vi "Teleop.vi"(10 "Match Info":T2={"Autonomous Elapsed Seconds"=0.0, "TeleOp Elapsed Seconds"=0.0, "Disabled Elapsed Seconds"=0.0, "Visited Autonomous"=FALSE, "Visited TeleOp"=FALSE, "Visited Disabled"=FALSE, "Autonomous Settings"={"Autonomous Style"=enum."Independent", "VI Refnum"=refnum}}, 11 "Call Context":T3) -> ()   [LabVIEW 2016]
doc: "This VI is called for each TeleOp packet received from the DS where the robot is not disabled. It is often used to read from the joysticks and update I/O or to update setpoints for timed control loops. It should complete and return within 20 milliseconds or it may miss DS packets."
uses:
  <vilib>/Rock Robotics/WPI/DriverStation/WPI_DriverStationDerivedRobotMode.ctl
  <vilib>/Rock Robotics/WPI/DriverStation/WPI_DriverStationMatch Info.ctl
  <vilib>/Rock Robotics/WPI/ThirdParty/CanMotor/TalonSRX/WPI_CANTalonSRX_GlobalStatus.ctl
  <vilib>/Rock Robotics/WPI/Relay/WPI_RelayValue.ctl
  <vilib>/Rock Robotics/Network Tables/NT Read Number.vi
  <vilib>/Rock Robotics/Network Tables/NT Read Boolean.vi
  <vilib>/Rock Robotics/WPI/Utilities/WPI_GetSetVariantRefNum.vi
  <vilib>/Rock Robotics/Network Tables/NT Write Boolean Array.vi
  <vilib>/Rock Robotics/Network Tables/NT Write Numeric Array.vi
  <vilib>/Rock Robotics/WPI/Ultrasonic/WPI_SonarMB1010DigitalRefNum Registry Get.vi
  <vilib>/Rock Robotics/WPI/Ultrasonic/WPI_SonarMB1010DigitalGetRange.vi
  <vilib>/Rock Robotics/Network Tables/NT Write Number.vi
  <vilib>/gmath/NI_Gmath.lvlib
panel:
  in  "Low Speed Divisor":dbl format="%#_13g"
  out "Encoder Position 2":dbl
  out "Talon SRX Status":T1
  out "Encoder Position":dbl
  in  "Positions":i32[](array[numeric])
  out "Angle":dbl format="%#_13g"
  in  "Control Effort":dbl[](array[numeric])=[0.0, 0.0, 0.0, 0.0]
  in  "RPM Array":dbl[](array[numeric])=[0.0, 0.0, 0.0, 0.0]
  out "Encoder Index Count":dbl
  in  "OR Speed":dbl
  in  "Override?":bool
  out "Shooter RPM":dbl
  in  "kP":dbl=1.0 format="%#_13g"
  out "Shooter RPM":dbl(graph)
  in  "SET RPM":dbl format="%#_13g"
  in  "Tab Control":enum32{"Page 1", "Page 2"}(tab)
  out "Shooter Current":dbl
  out "Shooter Current":dbl(graph)
  out "Distance":dbl
  out "Sample Slider 0":dbl(slide) scale=0.0..5.0
  out "Sample Boolean 1":bool
  out "Sample Boolean 0":bool
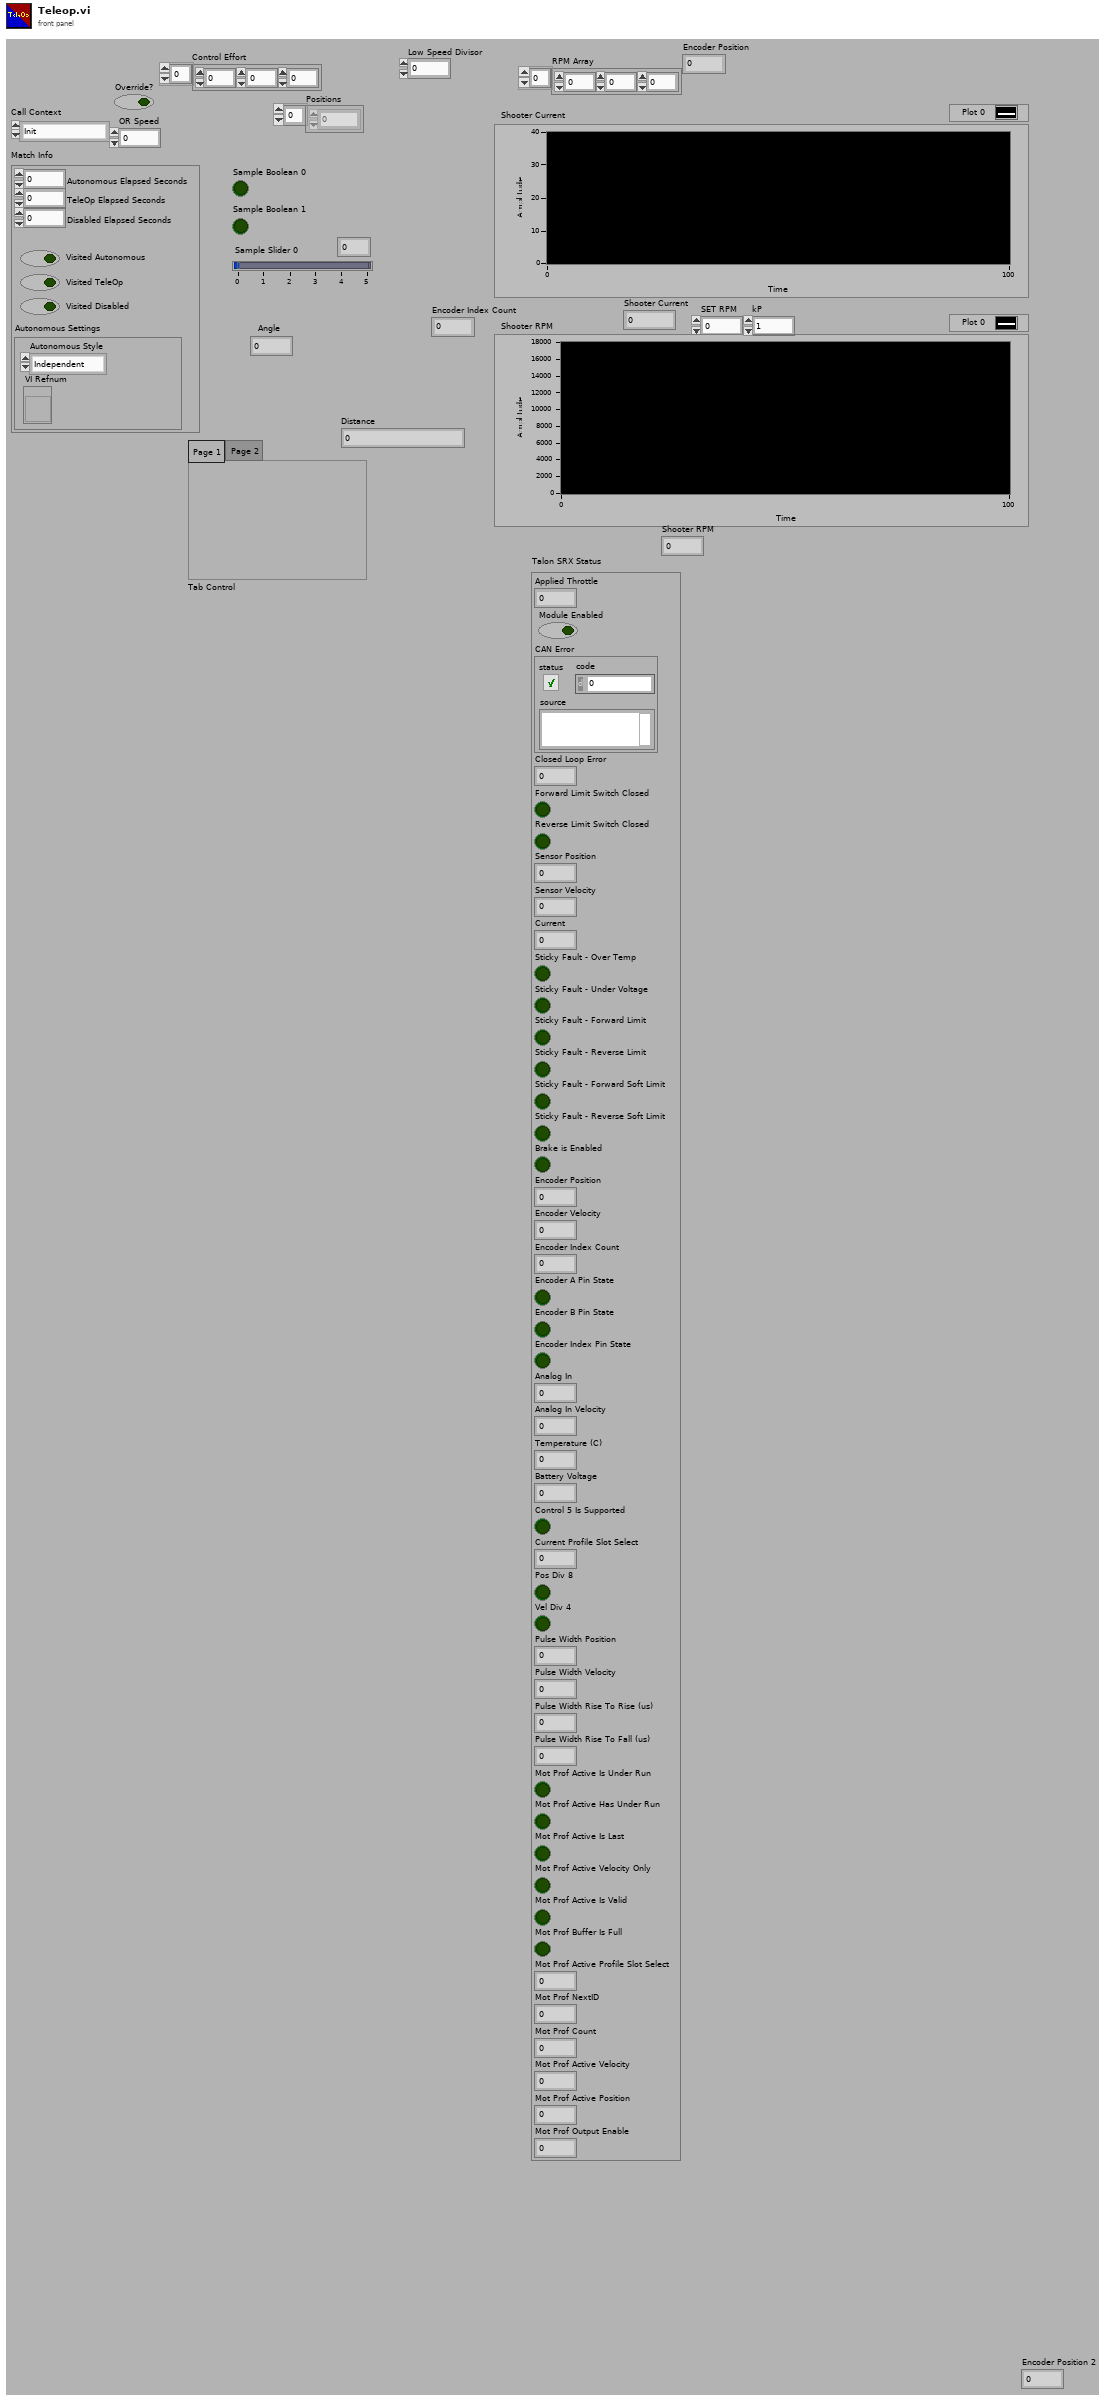
[diagram p1: front panel]
types:
  T1 = typedef "WPI_CANTalonSRX_GlobalStatus.ctl" = cluster{"Applied Throttle":dbl, "Module Enabled":bool, "CAN Error":errorcluster, "Closed Loop Error":dbl, "Forward Limit Switch Closed":bool, "Reverse Limit Switch Closed":bool, "Sensor Position":dbl, "Sensor Velocity":dbl, "Current":dbl, "Sticky Fault - Over Temp":bool, "Sticky Fault - Under Voltage":bool, "Sticky Fault - Forward Limit":bool, "Sticky Fault - Reverse Limit":bool, "Sticky Fault - Forward Soft Limit":bool, "Sticky Fault - Reverse Soft Limit":bool, "Brake is Enabled":bool, "Encoder Position":dbl, "Encoder Velocity":dbl, "Encoder Index Count":dbl, "Encoder A Pin State":bool, "Encoder B Pin State":bool, "Encoder Index Pin State":bool, "Analog In":dbl, "Analog In Velocity":dbl, "Temperature (C)":dbl, "Battery Voltage":dbl, "Control 5 Is Supported":bool, "Current Profile Slot Select":dbl, "Pos Div 8":bool, "Vel Div 4":bool, "Pulse Width Position":i32, "Pulse Width Velocity":i32, "Pulse Width Rise To Rise (us)":i32, "Pulse Width Rise To Fall (us)":i32, "Mot Prof Active Is Under Run":bool, "Mot Prof Active Has Under Run":bool, "Mot Prof Active Is Last":bool, "Mot Prof Active Velocity Only":bool, "Mot Prof Active Is Valid":bool, "Mot Prof Buffer Is Full":bool, "Mot Prof Active Profile Slot Select":i32, "Mot Prof NextID":i32, "Mot Prof Count":i32, "Mot Prof Active Velocity":dbl, "Mot Prof Active Position":dbl, "Mot Prof Output Enable":i32}
  T2 = typedef "WPI_DriverStationMatch Info.ctl" = cluster{"Autonomous Elapsed Seconds":dbl, "TeleOp Elapsed Seconds":dbl, "Disabled Elapsed Seconds":dbl, "Visited Autonomous":bool, "Visited TeleOp":bool, "Visited Disabled":bool, "Autonomous Settings":cluster{"Autonomous Style":enum16{"Iterative", "Independent"}, "VI Refnum":refnum<vi>}}
  T3 = typedef "WPI_DriverStationDerivedRobotMode.ctl" = enum16{"Init", "Execute", "Stop"}
  T4 = typedef "WPI_MotorControlDeviceRef.ctl" = cluster{"DeviceStatus":errorcluster, "Type":T5, "PWM":cluster{"PWM Channel":T6, "DeadBand":T7}, "CAN":cluster{"Device Number":u8, "SetOutput VI Ref":variant, "GetOutput VI Ref":variant, "Enable VI Ref":variant, "Disable VI Ref":variant, "Data":variant}, "Invert":bool}
  T5 = typedef "WPI_MotorControlType.ctl" = enum16{"PWM", "CAN"}
  T6 = typedef "FPGA_DIOPWMChannel.ctl" = enum8{"PWM 0", "PWM 1", "PWM 2", "PWM 3", "PWM 4", "PWM 5", "PWM 6", "PWM 7", "PWM 8", "PWM 9", "PWM MXP 0", "PWM MXP 1", "PWM MXP 2", "PWM MXP 3", "PWM MXP 4", "PWM MXP 5", "PWM MXP 6", "PWM MXP 7", "PWM MXP 8", "PWM MXP 9", "Invalid"}
  T7 = typedef "WPI_PWMDeadband.ctl" = cluster{"Name":string, "maxPositivePwm":i32, "minPositivePwm":i32, "centerPwm":i32, "maxNegativePwm":i32, "minNegativePwm":i32, "angularRange":u16}
  T8 = typedef "WPI_RelayValue.ctl" = enum16{"Off", "On", "Forward", "Reverse"}
  T9 = typedef "WPI_JoystickDevRef.ctl" = cluster{"Device":T10}
  T10 = typedef "WPI_JoystickDeviceEnum.ctl" = enum16{"USB 0", "USB 1", "USB 2", "USB 3", "USB 4", "USB 5"}
  T11 = typedef "WPI_RelayDevRef.ctl" = cluster{"DevStatus":errorcluster, "Relay Channel":T12, "Relay Direction":T13}
  T12 = typedef "FPGA_DIORelayChannel.ctl" = enum8{"Relay 0", "Relay 1", "Relay 2", "Relay 3", "Invalid"}
  T13 = typedef "WPI_RelayDirection.ctl" = enum16{"Both directions", "Forward only", "Reverse only"}
  T14 = typedef "WPI_SonarMB1010DigitalDeviceRef.ctl" = cluster{"CounterDevRef":T15, "Scaling factor (s/in)":dbl}
  T15 = typedef "WPI_CounterDevRef.ctl" = cluster{"DevStatus":errorcluster, "CntIndex":T16}
  T16 = typedef "FPGA_CounterCtrSystemIndex.ctl" = enum8{"Ctr 0", "Ctr 1", "Ctr 2", "Ctr 3", "Ctr 4", "Ctr 5", "Ctr 6", "Ctr 7", "Invalid"}
  T17 = typedef "WPI_GyroDevRef.ctl" = cluster{"DevStatus":errorcluster, "Analog Channel":T18, "Offset":dbl, "Gain (VoltsPerDegree/Second)":dbl, "Gyro Type":enum16{"Analog", "XRS450"}, "Handle":i32, "SPI Bus":T19, "Device Found":bool, "Sample Rate":dbl, "Calibrate On Open":bool}
  T18 = typedef "FPGA_AIChannel.ctl" = enum8{"AI 0", "AI 1", "AI 2", "AI 3", "AI MXP 0", "AI MXP 1", "AI MXP 2", "AI MXP 3", "Invalid"}
  T19 = typedef "spi_bus.ctl" = enum16{"SPI On-Board, CS0", "SPI On-Board, CS1", "SPI On-Board, CS2", "SPI On-Board, CS3", "SPI MXP", "Invalid"}
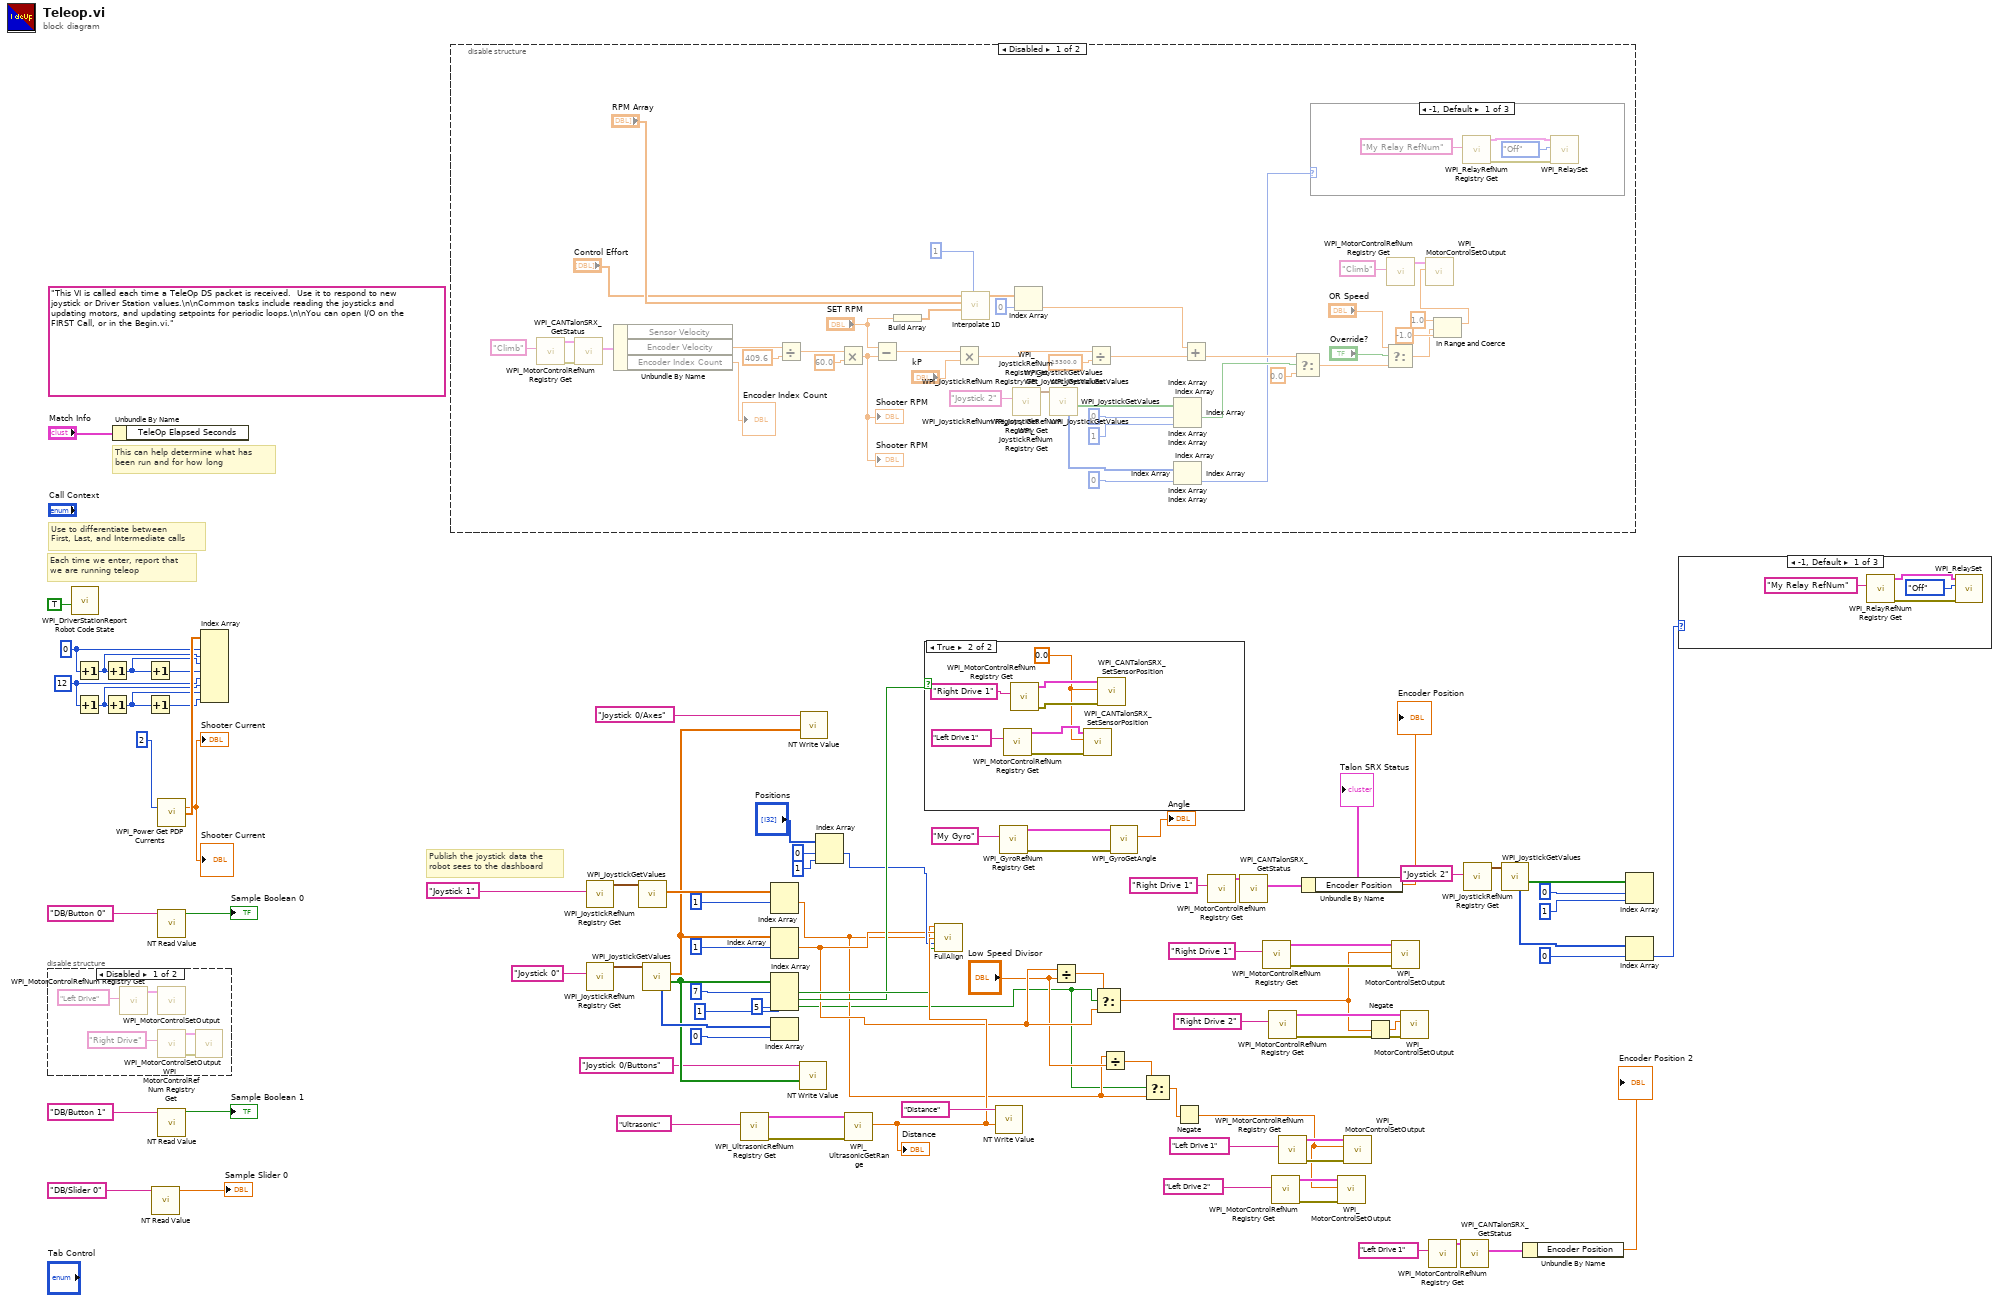
[diagram p0: block diagram]
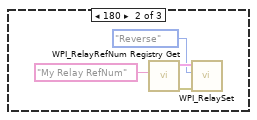
[diagram p2: hidden frame]
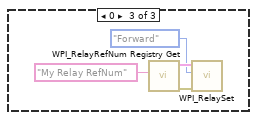
[diagram p3: hidden frame]
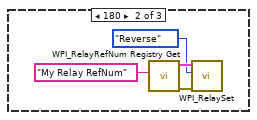
[diagram p5: hidden frame]
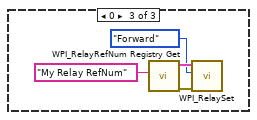
[diagram p6: hidden frame]
diagram:
  w79 = 12 ("PDP Channel")
  w83 = 0 ("PDP Channel")
  (unwired) "This VI is called each time a TeleOp DS packet is received.  Use it to respond to new joystick or Driver Station values.\n\nCommon tasks include reading the joysticks and updating motors, and updating setpoints for periodic loops.\n\nYou can open I/O on the FIRST Call, or in the Begin.vi."
  # "Publish the joystick data the\nrobot sees to the dashboard"
  # "Each time we enter, report that\nwe are running teleop"
  # "Use to differentiate between\nFirst, Last, and Intermediate calls"
  # "This can help determine what has\nbeen run and for how long"
  n1 = disable-structure shown="Disabled" {
    frame Disabled {
      n2 = call <vilib>:"WPI_MotorControlRefNum Registry Get.vi"("refnum name"="Left Drive") -> ("MotorControlDevRef"=w90:T4)  [unwired: 9 in, 1 out]
      n3 = call <vilib>:"WPI_MotorControlSetOutput.vi"("MotorControlDevRef"=w90) -> ()  [unwired: 8 in, 3 out]
      n4 = call <vilib>:"WPI_MotorControlRefNum Registry Get.vi"("refnum name"="Right Drive") -> ("error out"=w93:errorcluster, "MotorControlDevRef"=w92:T4)  [unwired: 9 in]
      n5 = call <vilib>:"WPI_MotorControlSetOutput.vi"("error in (no error)"=w93, "MotorControlDevRef"=w92) -> ()  [unwired: 7 in, 3 out]
    }
    frame Enabled {
    }
  }
  n6 = call <vilib>:"WPI_DriverStationReport Robot Code State.vi"("TeleOp"=TRUE ("Autonomous")) -> ()  [unwired: 10 in, 1 out]
  n7 = Increment(x=w83) -> (x+1=w82:i32)
  n8 = Increment(x=w79) -> (x+1=w78:i32)
  n9 = Increment(x=w82) -> (x+1=w80:i32)
  n10 = Increment(x=w78) -> (x+1=w76:i32)
  n11 = Unbundle By Name("Match Info") -> ()  [unwired: 1 out]
  n12 = Increment(x=w80) -> (x+1=w81:i32)
  n13 = Increment(x=w76) -> (x+1=w77:i32)
  n14 = call-poly <vilib>:"NT Read Value.vi"("Name"="DB/Slider 0" ("refnum name")) -> ("Numeric"=→"Sample Slider 0":dbl)  [unwired: 9 in, 1 out]
  n15 = call <vilib>:"WPI_Power Get PDP Currents.vi"("PDP Channel"=2) -> ("current (A)"=→"Shooter Current" →"Shooter Current":dbl, "all currents (A)"=w84:dbl[])  [unwired: 12 in, 1 out]
  n16 = call-poly <vilib>:"NT Read Value.vi"("Name"="DB/Button 0" ("refnum name")) -> ("Boolean"=→"Sample Boolean 0":bool)  [unwired: 9 in, 1 out]
  n17 = call-poly <vilib>:"NT Read Value.vi"("Name"="DB/Button 1" ("refnum name")) -> ("Boolean"=→"Sample Boolean 1":bool)  [unwired: 9 in, 1 out]
  n18 = Index Array(array=w84, index #1=w83, index #2=w82, index #3=w80, index #4=w81, index #5=w79, index #6=w78, index #7=w76, index #8=w77) -> ()  [unwired: 8 out]
  n19 = disable-structure shown="Disabled" {
    frame Disabled {
      n20 = call <vilib>:"WPI_MotorControlRefNum Registry Get.vi"("refnum name"="Climb") -> ("error out"=w114:errorcluster, "MotorControlDevRef"=w113:T4)  [unwired: 9 in]
      n21 = call <vilib>:"WPI_CANTalonSRX_GetStatus.vi"("error in (no error)"=w114, "CAN Talon SRX Ref"=w113) -> ("Talon SRX Status"=w123:T1)  [unwired: 7 in, 2 out]
      n22 = Unbundle By Name(w123) -> ("Encoder Velocity"=w117:dbl, "Encoder Index Count"=→"Encoder Index Count":dbl)  [unwired: 1 out]
      n23 = Divide(x=w117, y=409.6) -> (x/y=w116:dbl)
      n24 = Multiply(x=w116, y=60.0) -> (x*y=w119:dbl)
      "Shooter RPM" <- w119
      "Shooter RPM" <- w119
      n25 = Subtract(x="SET RPM", y=w119) -> (x-y=w104:dbl)
      n26 = Build Array("SET RPM") -> (w128:dbl[])
      n27 = Multiply(x=w104, y="kP") -> (x*y=w122:dbl)
      n28 = call <vilib>:"Interpolate 1D.vi"("method"=1, "xi"=w128, "X"="RPM Array", "Y"="Control Effort") -> ("yi"=w129:dbl[])  [unwired: 5 in, 2 out]
      n29 = call <vilib>:"WPI_JoystickRefNum Registry Get.vi"("refnum name"="Joystick 2") -> ("JoystickDevRef"=w163:T9)  [unwired: 1 in, 9 out]
      n30 = call <vilib>:"WPI_JoystickRefNum Registry Get.vi"("refnum name"="Joystick 2") -> ("JoystickDevRef"=w156:T9)  [unwired: 1 in, 9 out]
      n31 = call <vilib>:"WPI_JoystickRefNum Registry Get.vi"("refnum name"="Joystick 2") -> ("JoystickDevRef"=w145:T9)  [unwired: 1 in, 9 out]
      n32 = call <vilib>:"WPI_JoystickRefNum Registry Get.vi"("refnum name"="Joystick 2") -> ("JoystickDevRef"=w142:T9)  [unwired: 1 in, 9 out]
      n33 = call <vilib>:"WPI_JoystickRefNum Registry Get.vi"("refnum name"="Joystick 2") -> ("JoystickDevRef"=w99:T9)  [unwired: 1 in, 9 out]
      n34 = Index Array(array=w129, index=0) -> (element=w132:dbl)
      n35 = call <vilib>:"WPI_JoystickGetValues.vi"("JoystickDevRef"=w163) -> ("Buttons"=w161:bool[], "POVs"=w158:i16[])  [unwired: 6 in, 3 out]
      n36 = call <vilib>:"WPI_JoystickGetValues.vi"("JoystickDevRef"=w156) -> ("Buttons"=w154:bool[], "POVs"=w151:i16[])  [unwired: 6 in, 3 out]
      n37 = call <vilib>:"WPI_JoystickGetValues.vi"("JoystickDevRef"=w145) -> ("Buttons"=w147:bool[], "POVs"=w150:i16[])  [unwired: 6 in, 3 out]
      n38 = call <vilib>:"WPI_JoystickGetValues.vi"("JoystickDevRef"=w142) -> ("Buttons"=w140:bool[], "POVs"=w137:i16[])  [unwired: 6 in, 3 out]
      n39 = call <vilib>:"WPI_JoystickGetValues.vi"("JoystickDevRef"=w99) -> ("Buttons"=w101:bool[], "POVs"=w107:i16[])  [unwired: 6 in, 3 out]
      n40 = Divide(x=w122, y=15300.0) -> (x/y=w121:dbl)
      n41 = Index Array(array=w161, index #1=0 ("index"), index #2=1 ("index")) -> (element #1=w95:bool)  [unwired: 1 out]
      n42 = Index Array(array=w154, index #1=0 ("index"), index #2=1 ("index")) -> ()  [unwired: 2 out]
      n43 = Index Array(array=w147, index #1=0 ("index"), index #2=1 ("index")) -> ()  [unwired: 2 out]
      n44 = Index Array(array=w140, index #1=0 ("index"), index #2=1 ("index")) -> ()  [unwired: 2 out]
      n45 = Index Array(array=w101, index #1=0 ("index"), index #2=1 ("index")) -> ()  [unwired: 2 out]
      n46 = Index Array(array=w158, index=0) -> (element=w94:i16)
      n47 = Index Array(array=w151, index=0) -> ()  [unwired: 1 out]
      n48 = Index Array(array=w150, index=0) -> ()  [unwired: 1 out]
      n49 = Index Array(array=w137, index=0) -> ()  [unwired: 1 out]
      n50 = Index Array(array=w107, index=0) -> ()  [unwired: 1 out]
      n51 = Add(x=w132, y=w121) -> (x+y=w131:dbl)
      n52 = Select(t=w131, s=w95, f=0.0) -> (s? t:f=w111:dbl)
      n53 = case shown="-1, Default" w94 {
        frame -1, Default {
          n54 = call <vilib>:"WPI_RelayRefNum Registry Get.vi"("refnum name"="My Relay RefNum") -> ("error out"=w168:errorcluster, "RelayDevRef"=w167:T11)  [unwired: 9 in]
          n55 = call <vilib>:"WPI_RelaySet.vi"("error in (no error)"=w168, "RelayValue"=WPI_RelayValue."Off", "RelayDevRef"=w167) -> ()  [unwired: 7 in, 2 out]
        }
        frame 180 {
          n56 = call <vilib>:"WPI_RelayRefNum Registry Get.vi"("refnum name"="My Relay RefNum") -> ("error out"=w172:errorcluster, "RelayDevRef"=w171:T11)  [unwired: 9 in]
          n57 = call <vilib>:"WPI_RelaySet.vi"("error in (no error)"=w172, "RelayValue"=WPI_RelayValue."Reverse", "RelayDevRef"=w171) -> ()  [unwired: 7 in, 2 out]
        }
        frame 0 {
          n58 = call <vilib>:"WPI_RelayRefNum Registry Get.vi"("refnum name"="My Relay RefNum") -> ("error out"=w176:errorcluster, "RelayDevRef"=w175:T11)  [unwired: 9 in]
          n59 = call <vilib>:"WPI_RelaySet.vi"("error in (no error)"=w176, "RelayValue"=WPI_RelayValue."Forward", "RelayDevRef"=w175) -> ()  [unwired: 7 in, 2 out]
        }
      }
      n60 = Select(t="OR Speed", s="Override?", f=w111) -> (s? t:f=w133:dbl)
      n61 = call <vilib>:"WPI_MotorControlRefNum Registry Get.vi"("refnum name"="Climb") -> ("MotorControlDevRef"=w96:T4)  [unwired: 9 in, 1 out]
      n62 = In Range and Coerce(upper limit=1.0, x=w133, lower limit=-1.0) -> (coerced(x)=w136:dbl)  [unwired: 1 out]
      n63 = call <vilib>:"WPI_MotorControlSetOutput.vi"("Output"=w136, "MotorControlDevRef"=w96) -> ()  [unwired: 7 in, 3 out]
    }
    frame Enabled {
    }
  }
  n64 = call <vilib>:"WPI_JoystickRefNum Registry Get.vi"("refnum name"="Joystick 1") -> ("JoystickDevRef"=w55:T9)  [unwired: 1 in, 9 out]
  n65 = call <vilib>:"WPI_JoystickRefNum Registry Get.vi"("refnum name"="Joystick 0") -> ("JoystickDevRef"=w50:T9)  [unwired: 1 in, 9 out]
  n66 = call <vilib>:"WPI_JoystickGetValues.vi"("JoystickDevRef"=w55) -> ("Axes"=w54:dbl[])  [unwired: 6 in, 4 out]
  n67 = call <vilib>:"WPI_JoystickGetValues.vi"("JoystickDevRef"=w50) -> ("Buttons"=w63:bool[], "Axes"=w53:dbl[], "POVs"=w68:i16[])  [unwired: 6 in, 2 out]
  n68 = call-poly <vilib>:"WPI_UltrasonicRefNum Registry Get.vi"("refnum name"="Ultrasonic") -> ("error out"=w60:errorcluster, "SonarMB1010DigitalDevRef"=w61:T14)  [unwired: 9 in]
  n69 = Index Array(array=w54, index #1=1 ("index")) -> (element #1=w3:dbl)  [unwired: 1 in, 1 out]
  n70 = Index Array(array=w53, index #1=1 ("index")) -> (element #1=w8:dbl)  [unwired: 1 in, 1 out]
  n71 = Index Array(array=w63, index #1=7 ("index"), index #2=1, index #3=5 ("index")) -> (element #1=w38:bool, element #2=w36:bool, element #3=w2:bool)
  n72 = Index Array(array=w68, index=0) -> ()  [unwired: 1 out]
  n73 = call-poly <vilib>:"NT Write Value.vi"("Boolean Array"=w63, "Name"="Joystick 0/Buttons") -> ()  [unwired: 9 in, 1 out]
  n74 = call-poly <vilib>:"NT Write Value.vi"("Numeric Array"=w53, "Name"="Joystick 0/Axes") -> ()  [unwired: 9 in, 1 out]
  n75 = Index Array(array="Positions", index #1=0, index #2=1) -> (element #1=w32:i32)  [unwired: 1 out]
  n76 = call-poly <vilib>:"WPI_UltrasonicGetRange.vi"("error in"=w60, "SonarMB1010DigitalDevRef"=w61) -> ("Distance"=w39:dbl)  [unwired: 7 in, 2 out]
  "Distance" <- w39
  n77 = case shown="True" w36 {
    frame False {
    }
    frame True {
      w177 = 0.0 ("New Sensor Position")
      n78 = call <vilib>:"WPI_MotorControlRefNum Registry Get.vi"("refnum name"="Left Drive 1") -> ("error out"=w178:errorcluster, "MotorControlDevRef"=w179:T4)  [unwired: 9 in]
      n79 = call <vilib>:"WPI_MotorControlRefNum Registry Get.vi"("refnum name"="Right Drive 1") -> ("error out"=w181:errorcluster, "MotorControlDevRef"=w182:T4)  [unwired: 9 in]
      n80 = call <vilib>:"WPI_CANTalonSRX_SetSensorPosition.vi"("error in (no error)"=w178, "New Sensor Position"=w177, "CAN Talon SRX Ref"=w179) -> ()  [unwired: 7 in, 2 out]
      n81 = call <vilib>:"WPI_CANTalonSRX_SetSensorPosition.vi"("error in (no error)"=w181, "New Sensor Position"=w177, "CAN Talon SRX Ref"=w182) -> ()  [unwired: 7 in, 2 out]
    }
  }
  n82 = call "FullAlign.vi"("Joystick 0"=w3, "Joystick 1"=w8, "Distance"=w39, "Angle"=w32, "Button"=w38) -> ()  [unwired: 6 in, 5 out]
  n83 = call-poly <vilib>:"NT Write Value.vi"("Numeric"=w39, "Name"="Distance") -> ()  [unwired: 9 in, 1 out]
  n84 = call <vilib>:"WPI_GyroRefNum Registry Get.vi"("refnum name"="My Gyro") -> ("error out"=w67:errorcluster, "GyroDevRef"=w66:T17)  [unwired: 9 in]
  n85 = Divide(x=w8, y="Low Speed Divisor") -> (x/y=w7:dbl)
  n86 = Select(t=w7, s=w2, f=w8) -> (s? t:f=w6:dbl)
  n87 = Divide(x=w3, y="Low Speed Divisor") -> (x/y=w5:dbl)
  n88 = call <vilib>:"WPI_GyroGetAngle.vi"("error in"=w67, "GyroDevRef"=w66) -> ("Angle"=→"Angle":dbl)  [unwired: 5 in, 4 out]
  n89 = Select(t=w5, s=w2, f=w3) -> (s? t:f=w1:dbl)
  n90 = Negate(x=w1) -> (-x=w18:dbl)
  n91 = call <vilib>:"WPI_MotorControlRefNum Registry Get.vi"("refnum name"="Right Drive 1") -> ("MotorControlDevRef"=w16:T4)  [unwired: 9 in, 1 out]
  n92 = call <vilib>:"WPI_CANTalonSRX_GetStatus.vi"("CAN Talon SRX Ref"=w16) -> ("Talon SRX Status"=w17:T1)  [unwired: 8 in, 2 out]
  "Talon SRX Status" <- w17
  n93 = call <vilib>:"WPI_MotorControlRefNum Registry Get.vi"("refnum name"="Right Drive 1") -> ("error out"=w26:errorcluster, "MotorControlDevRef"=w27:T4)  [unwired: 9 in]
  n94 = call <vilib>:"WPI_MotorControlRefNum Registry Get.vi"("refnum name"="Right Drive 2") -> ("error out"=w31:errorcluster, "MotorControlDevRef"=w30:T4)  [unwired: 9 in]
  n95 = call <vilib>:"WPI_MotorControlRefNum Registry Get.vi"("refnum name"="Left Drive 2") -> ("error out"=w23:errorcluster, "MotorControlDevRef"=w24:T4)  [unwired: 9 in]
  n96 = call <vilib>:"WPI_MotorControlRefNum Registry Get.vi"("refnum name"="Left Drive 1") -> ("error out"=w20:errorcluster, "MotorControlDevRef"=w21:T4)  [unwired: 9 in]
  n97 = Unbundle By Name(w17) -> ("Encoder Position"=→"Encoder Position":dbl)
  n98 = call <vilib>:"WPI_MotorControlSetOutput.vi"("error in (no error)"=w23, "Output"=w18, "MotorControlDevRef"=w24) -> ()  [unwired: 6 in, 3 out]
  n99 = call <vilib>:"WPI_MotorControlSetOutput.vi"("error in (no error)"=w20, "Output"=w18, "MotorControlDevRef"=w21) -> ()  [unwired: 6 in, 3 out]
  n100 = Negate(x=w6) -> (-x=w19:dbl)
  n101 = call <vilib>:"WPI_MotorControlSetOutput.vi"("error in (no error)"=w26, "Output"=w6, "MotorControlDevRef"=w27) -> ()  [unwired: 6 in, 3 out]
  n102 = call <vilib>:"WPI_MotorControlSetOutput.vi"("error in (no error)"=w31, "Output"=w19, "MotorControlDevRef"=w30) -> ()  [unwired: 6 in, 3 out]
  n103 = call <vilib>:"WPI_MotorControlRefNum Registry Get.vi"("refnum name"="Left Drive 1") -> ("MotorControlDevRef"=w10:T4)  [unwired: 9 in, 1 out]
  n104 = call <vilib>:"WPI_CANTalonSRX_GetStatus.vi"("CAN Talon SRX Ref"=w10) -> ("Talon SRX Status"=w13:T1)  [unwired: 8 in, 2 out]
  n105 = call <vilib>:"WPI_JoystickRefNum Registry Get.vi"("refnum name"="Joystick 2") -> ("JoystickDevRef"=w43:T9)  [unwired: 1 in, 9 out]
  n106 = call <vilib>:"WPI_JoystickGetValues.vi"("JoystickDevRef"=w43) -> ("Buttons"=w45:bool[], "POVs"=w48:i16[])  [unwired: 6 in, 3 out]
  n107 = Unbundle By Name(w13) -> ("Encoder Position"=→"Encoder Position 2":dbl)
  n108 = Index Array(array=w45, index #1=0 ("index"), index #2=1 ("index")) -> ()  [unwired: 2 out]
  n109 = Index Array(array=w48, index=0) -> (element=w41:i16)
  n110 = case shown="-1, Default" w41 {
    frame -1, Default {
      n111 = call <vilib>:"WPI_RelayRefNum Registry Get.vi"("refnum name"="My Relay RefNum") -> ("error out"=w187:errorcluster, "RelayDevRef"=w186:T11)  [unwired: 9 in]
      n112 = call <vilib>:"WPI_RelaySet.vi"("error in (no error)"=w187, "RelayValue"=WPI_RelayValue."Off", "RelayDevRef"=w186) -> ()  [unwired: 7 in, 2 out]
    }
    frame 180 {
      n113 = call <vilib>:"WPI_RelayRefNum Registry Get.vi"("refnum name"="My Relay RefNum") -> ("error out"=w191:errorcluster, "RelayDevRef"=w190:T11)  [unwired: 9 in]
      n114 = call <vilib>:"WPI_RelaySet.vi"("error in (no error)"=w191, "RelayValue"=WPI_RelayValue."Reverse", "RelayDevRef"=w190) -> ()  [unwired: 7 in, 2 out]
    }
    frame 0 {
      n115 = call <vilib>:"WPI_RelayRefNum Registry Get.vi"("refnum name"="My Relay RefNum") -> ("error out"=w195:errorcluster, "RelayDevRef"=w194:T11)  [unwired: 9 in]
      n116 = call <vilib>:"WPI_RelaySet.vi"("error in (no error)"=w195, "RelayValue"=WPI_RelayValue."Forward", "RelayDevRef"=w194) -> ()  [unwired: 7 in, 2 out]
    }
  }
